vi "Lab Panel V5.10.vi"() -> ()   [LabVIEW 2013] (continued)
              n217 = Bundle By Name(cluster=w250, "TL-1"=w242, "TN-1"=w241, "TL-2"=w240, "TN-2"=w239, "TL -1COUNT"=w247, "TN-1 COUNT"=w247, "TL-2 COUNT"=w247, "TN-2 COUNT"=w247) -> (w248:T9)
              n218 = Bundle(cluster=w245, "Tmp Live"=w240, "Tmp Neut"=w239) -> (w243:T2)  [unwired: 3 in]
              n219 = Bundle(cluster=w246, "Tmp Live"=w242, "Tmp Neut"=w241) -> (w244:T2)  [unwired: 3 in]
              n220 = local write "TEMP LA02"(w248) -> ()
              n221 = local write "SIG LAB02-1"(w244) -> ()
              n222 = local write "SIG LAB02-2"(w243) -> ()
            }
            frame #4 {
              w259 = 0
              n223 = local read "LAB03 TEMP"() -> (w261:T12)
              n224 = Unbundle By Name(w261) -> ("T1 Live"=w254:dbl, "T1 Neut"=w253:dbl, "T2 Live"=w252:dbl, "T2 Neut"=w251:dbl)  [unwired: 2 out]
              n225 = local read "SIG LAB03-1"() -> (w258:T2)
              n226 = local read "SIG LAB03-2"() -> (w257:T2)
              n227 = local read "TEMP LA03"() -> (w262:T9)
              n228 = Bundle By Name(cluster=w262, "TL-1"=w254, "TN-1"=w253, "TL-2"=w252, "TN-2"=w251, "TL -1COUNT"=w259, "TN-1 COUNT"=w259, "TL-2 COUNT"=w259, "TN-2 COUNT"=w259) -> (w260:T9)
              n229 = Bundle(cluster=w257, "Tmp Live"=w252, "Tmp Neut"=w251) -> (w255:T2)  [unwired: 3 in]
              n230 = Bundle(cluster=w258, "Tmp Live"=w254, "Tmp Neut"=w253) -> (w256:T2)  [unwired: 3 in]
              n231 = local write "TEMP LA03"(w260) -> ()
              n232 = local write "SIG LAB03-2"(w255) -> ()
              n233 = local write "SIG LAB03-1"(w256) -> ()
            }
            frame #5 {
              w271 = 0
              n234 = local read "LAB04 TEMP"() -> (w273:T12)
              n235 = Unbundle By Name(w273) -> ("T1 Live"=w266:dbl, "T1 Neut"=w265:dbl, "T2 Live"=w264:dbl, "T2 Neut"=w263:dbl)  [unwired: 2 out]
              n236 = local read "SIG LAB04-2"() -> (w269:T2)
              n237 = local read "SIG LAB04-1"() -> (w270:T2)
              n238 = local read "TEMP LA04"() -> (w274:T9)
              n239 = Bundle By Name(cluster=w274, "TL-1"=w266, "TN-1"=w265, "TL-2"=w264, "TN-2"=w263, "TL -1COUNT"=w271, "TN-1 COUNT"=w271, "TL-2 COUNT"=w271, "TN-2 COUNT"=w271) -> (w272:T9)
              n240 = Bundle(cluster=w269, "Tmp Live"=w264, "Tmp Neut"=w263) -> (w267:T2)  [unwired: 3 in]
              n241 = Bundle(cluster=w270, "Tmp Live"=w266, "Tmp Neut"=w265) -> (w268:T2)  [unwired: 3 in]
              n242 = local write "SIG LAB04-2"(w267) -> ()
              n243 = local write "TEMP LA04"(w272) -> ()
              n244 = local write "SIG LAB04-1"(w268) -> ()
            }
            frame #6 {
              w283 = 0
              n245 = local read "LAB05 TEMP"() -> (w285:T12)
              n246 = Unbundle By Name(w285) -> ("T1 Live"=w278:dbl, "T1 Neut"=w277:dbl, "T2 Live"=w276:dbl, "T2 Neut"=w275:dbl)  [unwired: 2 out]
              n247 = local read "SIG LAB05-2"() -> (w281:T2)
              n248 = local read "SIG LAB05-1"() -> (w282:T2)
              n249 = local read "TEMP LA05"() -> (w286:T9)
              n250 = Bundle By Name(cluster=w286, "TL-1"=w278, "TN-1"=w277, "TL-2"=w276, "TN-2"=w275, "TL -1COUNT"=w283, "TN-1 COUNT"=w283, "TL-2 COUNT"=w283, "TN-2 COUNT"=w283) -> (w284:T9)
              n251 = Bundle(cluster=w281, "Tmp Live"=w276, "Tmp Neut"=w275) -> (w279:T2)  [unwired: 3 in]
              n252 = Bundle(cluster=w282, "Tmp Live"=w278, "Tmp Neut"=w277) -> (w280:T2)  [unwired: 3 in]
              n253 = local write "SIG LAB05-2"(w279) -> ()
              n254 = local write "SIG LAB05-1"(w280) -> ()
              n255 = local write "TEMP LA05"(w284) -> ()
            }
          }
        }
        frame #8 {
          # "enable front panel, all settings done"
          n256 = property on="Tab Control 2" class="TabCtl (strict)"("DisabledEnum"=T16."Enabled" ("Disabled")) -> ()  [unwired: 2 in, 2 out]
          n257 = property on="Tab Control 2" class="TabCtl (strict)"("Value"=0) -> ()  [unwired: 2 in, 2 out]
        }
        frame #9 {
          n258 = property on="Tab Control 2" class="TabCtl (strict)"("Value"=0) -> ()  [unwired: 2 in, 2 out]
        }
      }
    }
    frame #2 {
      n259 = node-c288("loop  delay(mS)") -> (w292:T17)  [unwired: 3 in]
      n260 = timed-loop {
        timing: w292 -> [_]
        timing-out: [_] -> w291
        i -> [w314]
        stop <- "stop" stop-if-true
        n261 = node-c288() -> ()  [unwired: 1 in, 1 out]
        n262 = global write "Global display 1.vi" "stop disp"("stop") -> ()
        n263 = local read "SELECT LAB05-2"() -> (w294:T3)
        n264 = local read "SELECT LAB05-1"() -> (w295:T3)
        n265 = local read "SELECT LAB04-2"() -> (w296:T3)
        n266 = local read "SELECT LAB03-1"() -> (w299:T3)
        n267 = local read "SELECT LAB02-2"() -> (w300:T3)
        n268 = local read "SELECT LAB01-1"() -> (w303:T3)
        n269 = local read "SELECT LAB03-2"() -> (w298:T3)
        n270 = local read "SELECT LAB01-2"() -> (w302:T3)
        n271 = local read "SELECT LAB04-1"() -> (w297:T3)
        n272 = local read "SELECT LAB02-1"() -> (w301:T3)
        n273 = local read "run lab03-2"() -> (w308:bool)
        n274 = local read "run lab04-1"() -> (w307:bool)
        n275 = local read "run lab05-1"() -> (w305:bool)
        n276 = local read "run lab04-2"() -> (w306:bool)
        n277 = local read "run lab05-2"() -> (w304:bool)
        n278 = local read "run lab03-1"() -> (w309:bool)
        n279 = local read "run lab02-2"() -> (w310:bool)
        n280 = local read "run lab02-1"() -> (w311:bool)
        n281 = local read "run lab01-1"() -> (w313:bool)
        n282 = local read "run lab01-2"() -> (w312:bool)
        n283 = stacked-sequence {
          seq-local: [_ w379 _ _ _ _ _ _ _ _ _ _ _ _ _ _ _ _ _ _ _ _ _] -> [_ _ _ _ _ w2480 _ _ _ _ _ _ _ _ _ _ _ _ _ _ _ _ _]
          seq-local: [_ w378 _ _ _ _ _ _ _ _ _ _ _ _ _ _ _ _ _ _ _ _ _] -> [_ _ _ _ _ w2479 _ _ _ _ _ _ _ _ _ _ _ _ _ _ _ _ _]
          seq-local: [_ w365 _ _ _ _ _ _ _ _ _ _ _ _ _ _ _ _ _ _ _ _ _] -> [_ _ _ _ _ w2478 _ _ _ _ _ _ _ _ _ _ _ _ _ _ _ _ _]
          seq-local: [_ w364 _ _ _ _ _ _ _ _ _ _ _ _ _ _ _ _ _ _ _ _ _] -> [_ _ _ _ _ w2477 _ _ _ _ _ _ _ _ _ _ _ _ _ _ _ _ _]
          seq-local: [_ w363 _ _ _ _ _ _ _ _ _ _ _ _ _ _ _ _ _ _ _ _ _] -> [_ _ _ _ _ w2476 _ _ _ _ _ _ _ _ _ _ _ _ _ _ _ _ _]
          seq-local: [_ w362 _ _ _ _ _ _ _ _ _ _ _ _ _ _ _ _ _ _ _ _ _] -> [_ _ _ _ _ w2475 _ _ _ _ _ _ _ _ _ _ _ _ _ _ _ _ _]
          seq-local: [_ w361 _ _ _ _ _ _ _ _ _ _ _ _ _ _ _ _ _ _ _ _ _] -> [_ _ _ _ _ w2474 _ _ _ _ _ _ _ _ _ _ _ _ _ _ _ _ _]
          seq-local: [_ w360 _ _ _ _ _ _ _ _ _ _ _ _ _ _ _ _ _ _ _ _ _] -> [_ _ _ _ _ w2473 _ _ _ _ _ _ _ _ _ _ _ _ _ _ _ _ _]
          seq-local: [_ w359 _ _ _ _ _ _ _ _ _ _ _ _ _ _ _ _ _ _ _ _ _] -> [_ _ _ _ _ w2472 _ _ _ _ _ _ _ _ _ _ _ _ _ _ _ _ _]
          seq-local: [_ w358 _ _ _ _ _ _ _ _ _ _ _ _ _ _ _ _ _ _ _ _ _] -> [_ _ _ _ _ w2471 _ _ _ _ _ _ _ _ _ _ _ _ _ _ _ _ _]
          tunnel: w313 -> [_ _ w395 w643 w2070 w2500 w2815 w3302 _ _ _ _ w3790 _ w4747 _ _ w5034 w5337 w5519 _ _ _]
          tunnel: w312 -> [_ _ w394 w641 w2069 w2499 w2816 w3301 _ _ _ _ w3789 _ w4745 _ _ w5033 w5336 w5517 _ _ _]
          tunnel: w311 -> [_ _ w393 w639 w2068 w2498 w2814 w3300 _ _ _ _ w3788 _ w4743 _ _ w5032 w5335 w5516 _ _ _]
          tunnel: w310 -> [_ _ w392 w637 w2067 w2497 w2813 w3299 _ _ _ _ w3787 _ w4741 _ _ w5031 w5334 w5515 _ _ _]
          tunnel: w309 -> [_ _ w391 w635 w2066 w2496 w2812 w3298 _ _ _ _ w3786 _ w4739 _ _ w5030 w5333 w5514 _ _ _]
          tunnel: w308 -> [_ _ w390 w633 w2065 w2495 w2811 w3297 _ _ _ _ w3785 _ w4737 _ _ w5029 w5332 w5513 _ _ _]
          tunnel: w307 -> [_ _ w389 w631 w2064 w2494 w2810 w3296 _ _ _ _ w3784 _ w4735 _ _ w5028 w5331 w5512 _ _ _]
          tunnel: w306 -> [_ _ w388 w629 w2063 w2493 w2809 w3295 _ _ _ _ w3783 _ w4733 _ _ w5027 w5330 w5511 _ _ _]
          tunnel: w305 -> [_ _ w387 w627 w2062 w2492 w2808 w3294 _ _ _ _ w3782 _ w4731 _ _ w5026 w5329 w5510 _ _ _]
          tunnel: w304 -> [_ _ w386 w625 w2061 w2491 w2807 w3293 _ _ _ _ w3781 _ w4729 _ _ w5025 w5328 w5509 _ _ _]
          tunnel: w303 -> [_ _ _ w642 w2060 w2490 _ _ _ _ _ _ _ _ w4749 _ _ _ _ _ w5863 _ _]
          tunnel: w302 -> [_ _ _ w640 w2059 w2489 _ _ _ _ _ _ _ _ w4744 _ _ _ _ _ w5862 _ _]
          tunnel: w301 -> [_ _ _ w638 w2058 w2488 _ _ _ _ _ _ _ _ w4742 _ _ _ _ _ w5861 _ _]
          tunnel: w300 -> [_ _ _ w636 w2057 w2487 _ _ _ _ _ _ _ _ w4740 _ _ _ _ _ w5860 _ _]
          tunnel: w299 -> [_ _ _ w634 w2056 w2486 _ _ _ _ _ _ _ _ w4738 _ _ _ _ _ w5859 _ _]
          tunnel: w298 -> [_ _ _ w632 w2055 w2485 _ _ _ _ _ _ _ _ w4736 _ _ _ _ _ w5858 _ _]
          tunnel: w297 -> [_ _ _ w630 w2054 w2484 _ _ _ _ _ _ _ _ w4734 _ _ _ _ _ w5857 _ _]
          tunnel: w296 -> [_ _ _ w628 w2053 w2483 _ _ _ _ _ _ _ _ w4732 _ _ _ _ _ w5856 _ _]
          tunnel: w295 -> [_ _ _ w626 w2052 w2482 _ _ _ _ _ _ _ _ w4730 _ _ _ _ _ w5855 _ _]
          tunnel: w294 -> [_ _ _ w624 w2051 w2481 _ _ _ _ _ _ _ _ w4728 _ _ _ _ _ w5854 _ _]
          frame #0 {
            w321 = FALSE
            w326 = 0.5
            # "set up cycle control"
            n284 = local read "jig cycle"() -> (w325:dbl)
            n285 = local read "Amps Fail level"() -> (w319:dbl)
            n286 = Divide(x="JIG ON TIME (S)", y=w326) -> (x/y=→"on loops":dbl)
            n287 = Divide(x="JIG OFF TIME (S)", y=w326) -> (x/y=→"off loops":dbl)
            n288 = global write "Global display 3.vi" "Amps Fail"(w319) -> ()
            n289 = Increment(x=w325) -> (x+1=w324:dbl)
            n290 = local write "TEMP"(w321) -> ()
            n291 = local write "AI"(w321) -> ()
            n292 = local read "Network Directory"() -> (w318:path)
            n293 = local write "jig cycle"(w324) -> ()
            n294 = call "sub vi - check network dir v2.vi"("PATH"=w318) -> ("error"=w317:bool)  [unwired: 10 in]
            n295 = local write "network error"(w317) -> ()
            n296 = global write "Global display 3.vi" "network drive"(w317) -> ()
            n297 = event shown="[1] \"ADMIN\": Value Change" {
              selector: _ -> [_ _]
              dyn-events: _ -> [_ _]
              timeout: 10 -> [_ _]
              event Timeout {
                n298 = event-data() -> ()  [unwired: 1 in, 3 out]
              }
              event "ADMIN": Value Change {
                n299 = event-data() -> ()  [unwired: 1 in, 6 out]
                n300 = stacked-sequence {
                  seq-local: [_ w330 _] -> [_ _ w331]
                  frame #0 {
                    n301 = global write "Global 1.vi" "password"("9949") -> ()
                  }
                  frame #1 {
                    n302 = call "sub vi - password 1.vi"() -> ("RESULT"=w330:bool)  [unwired: 11 in]
                  }
                  frame #2 {
                    w333 = FALSE
                    n303 = property on="Tab Control 2" class="TabCtl (strict)"() -> ("Pages"=w337:refnum<vi>[])  [unwired: 2 in, 2 out]
                    n304 = Select(t=TRUE, s=w331, f=w333) -> (s? t:f=w332:bool)
                    n305 = Index Array(array=w337, index=8) -> (element=w335:refnum<vi>)
                    n306 = property class="Page"(reference=w335, "PageVis"=w332) -> ()  [unwired: 1 in, 2 out]
                    n307 = local write "ADMIN"(w333) -> ()
                  }
                }
              }
            }
          }
          frame #1 {
            w375 = 60.0
            # "convert temperature rise minutes to cycles"
            n308 = local read "SET LAB05-2"() -> (w339:T5)
            n309 = local read "SET LAB05-1"() -> (w341:T5)
            n310 = local read "SET LAB04-2"() -> (w343:T5)
            n311 = local read "SET LAB01-1"() -> (w357:T5)
            n312 = local read "SET LAB01-2"() -> (w355:T5)
            n313 = local read "SET LAB02-2"() -> (w351:T5)
            n314 = local read "SET LAB04-1"() -> (w345:T5)
            n315 = local read "SET LAB03-1"() -> (w349:T5)
            n316 = local read "SET LAB03-2"() -> (w347:T5)
            n317 = local read "SET LAB02-1"() -> (w353:T5)
            n318 = local read "JIG OFF TIME (S)"() -> (w380:dbl)
            n319 = local read "JIG ON TIME (S)"() -> (w381:dbl)
            n320 = Unbundle(w339) -> ("T-RISE mins"=w338:dbl)  [unwired: 4 out]
            n321 = Unbundle(w341) -> ("T-RISE mins"=w340:dbl)  [unwired: 4 out]
            n322 = Unbundle(w357) -> ("T-RISE mins"=w356:dbl)  [unwired: 4 out]
            n323 = Unbundle(w343) -> ("T-RISE mins"=w342:dbl)  [unwired: 4 out]
            n324 = Unbundle(w355) -> ("T-RISE mins"=w354:dbl)  [unwired: 4 out]
            n325 = Unbundle(w353) -> ("T-RISE mins"=w352:dbl)  [unwired: 4 out]
            n326 = Unbundle(w345) -> ("T-RISE mins"=w344:dbl)  [unwired: 4 out]
            n327 = Unbundle(w351) -> ("T-RISE mins"=w350:dbl)  [unwired: 4 out]
            n328 = Unbundle(w347) -> ("T-RISE mins"=w346:dbl)  [unwired: 4 out]
            n329 = Unbundle(w349) -> ("T-RISE mins"=w348:dbl)  [unwired: 4 out]
            n330 = Add(x=w381, y=w380) -> (x+y=w374:dbl)
            n331 = Multiply(x=w375, y=w346) -> (x*y=w370:dbl)
            n332 = Multiply(x=w375, y=w344) -> (x*y=w369:dbl)
            n333 = Multiply(x=w375, y=w342) -> (x*y=w368:dbl)
            n334 = Multiply(x=w375, y=w340) -> (x*y=w367:dbl)
            n335 = Multiply(x=w375, y=w338) -> (x*y=w366:dbl)
            n336 = Multiply(x=w375, y=w354) -> (x*y=w376:dbl)
            n337 = Multiply(x=w375, y=w348) -> (x*y=w371:dbl)
            n338 = Multiply(x=w375, y=w356) -> (x*y=w377:dbl)
            n339 = Multiply(x=w375, y=w352) -> (x*y=w373:dbl)
            n340 = Multiply(x=w375, y=w350) -> (x*y=w372:dbl)
            n341 = Divide(x=w367, y=w374) -> (x/y=w359:dbl)
            n342 = Divide(x=w368, y=w374) -> (x/y=w360:dbl)
            n343 = Divide(x=w369, y=w374) -> (x/y=w361:dbl)
            n344 = Divide(x=w366, y=w374) -> (x/y=w358:dbl)
            n345 = Divide(x=w371, y=w374) -> (x/y=w363:dbl)
            n346 = Divide(x=w377, y=w374) -> (x/y=w379:dbl)
            n347 = Divide(x=w376, y=w374) -> (x/y=w378:dbl)
            n348 = Divide(x=w373, y=w374) -> (x/y=w365:dbl)
            n349 = Divide(x=w372, y=w374) -> (x/y=w364:dbl)
            n350 = Divide(x=w370, y=w374) -> (x/y=w362:dbl)
          }
          frame #2 {
            # "control cycle loops"
            n351 = local read "JIG OFF TIME (S)"() -> (w384:dbl)
            n352 = local read "JIG ON TIME (S)"() -> (w383:dbl)
            n353 = local read "jig cycle"() -> (w397:dbl)
            n354 = local read "on loops"() -> (w399:dbl)
            n355 = local read "off loops"() -> (w398:dbl)
            n356 = Add(x=w384, y=w383) -> (x+y=w382:dbl)
            n357 = Add(x=w399, y=w398) -> (x+y=w385:dbl)
            n358 = Greater Or Equal?(x=w397, y=w385) -> (x >= y?=w396:bool)
            n359 = case shown="True" w396 {
              tunnel: w395 -> [_ w433]
              tunnel: w394 -> [_ w432]
              tunnel: w393 -> [_ w431]
              tunnel: w392 -> [_ w430]
              tunnel: w391 -> [_ w429]
              tunnel: w390 -> [_ w428]
              tunnel: w389 -> [_ w427]
              tunnel: w388 -> [_ w426]
              tunnel: w387 -> [_ w425]
              tunnel: w386 -> [_ w424]
              tunnel: w382 -> [_ w423]
              frame False {
              }
              frame True {
                # "increment cycle value and convert cycles to minutes for temp rise"
                n360 = stacked-sequence {
                  frame #0 {
                    n361 = local read "Panel #"() -> (w436:dbl)
                    n362 = Increment(x=w436) -> (x+1=w435:dbl)
                    n363 = local write "Panel #"(w435) -> ()
                  }
                  frame #1 {
                    n364 = local read "Panel #"() -> (w437:dbl)
                    n365 = Greater?(x=w437, y=5) -> (0:w439:bool)
                    n366 = case shown="True" w439 {
                      frame False {
                      }
                      frame True {
                        n367 = local write "Panel #"(1) -> ()
                      }
                    }
                  }
                }
                n368 = local read "JIG RELAY CYCLES"() -> (w422:T8)
                n369 = local read "Panel #"() -> (→"Tp Ut":dbl)
                n370 = Unbundle By Name(w422) -> ("LAB01-1"=w420:dbl, "LAB01-2"=w418:dbl, "LAB02-1"=w416:dbl, "LAB02-2"=w414:dbl, "LAB03-1"=w412:dbl, "LAB03-2"=w410:dbl, "LAB04-1"=w408:dbl, "LAB04-2"=w406:dbl, "LAB05-1"=w404:dbl, "LAB05-2"=w402:dbl)
                n371 = stacked-sequence {
                  tunnel: w433 -> [w451 _ _ _ _ _ _ _ _ _]
                  tunnel: w432 -> [_ w468 _ _ _ _ _ _ _ _]
                  tunnel: w431 -> [_ _ w485 _ _ _ _ _ _ _]
                  tunnel: w430 -> [_ _ _ w502 _ _ _ _ _ _]
                  tunnel: w429 -> [_ _ _ _ w519 _ _ _ _ _]
                  tunnel: w428 -> [_ _ _ _ _ w536 _ _ _ _]
                  tunnel: w427 -> [_ _ _ _ _ _ w553 _ _ _]
                  tunnel: w426 -> [_ _ _ _ _ _ _ w570 _ _]
                  tunnel: w425 -> [_ _ _ _ _ _ _ _ w587 _]
                  tunnel: w424 -> [_ _ _ _ _ _ _ _ _ w604]
                  tunnel: w423 -> [w448 w465 w482 w499 w516 w533 w550 w567 w584 w601]
                  tunnel: w420 -> [w442 _ _ _ _ _ _ _ _ _]
                  tunnel: [w441 _ _ _ _ _ _ _ _ _] -> w419
                  tunnel: w418 -> [_ w459 _ _ _ _ _ _ _ _]
                  tunnel: [_ w458 _ _ _ _ _ _ _ _] -> w417
                  tunnel: w416 -> [_ _ w476 _ _ _ _ _ _ _]
                  tunnel: [_ _ w475 _ _ _ _ _ _ _] -> w415
                  tunnel: w414 -> [_ _ _ w493 _ _ _ _ _ _]
                  tunnel: [_ _ _ w492 _ _ _ _ _ _] -> w413
                  tunnel: w412 -> [_ _ _ _ w510 _ _ _ _ _]
                  tunnel: [_ _ _ _ w509 _ _ _ _ _] -> w411
                  tunnel: w410 -> [_ _ _ _ _ w527 _ _ _ _]
                  tunnel: [_ _ _ _ _ w526 _ _ _ _] -> w409
                  tunnel: w408 -> [_ _ _ _ _ _ w544 _ _ _]
                  tunnel: [_ _ _ _ _ _ w543 _ _ _] -> w407
                  tunnel: w406 -> [_ _ _ _ _ _ _ w561 _ _]
                  tunnel: [_ _ _ _ _ _ _ w560 _ _] -> w405
                  tunnel: w404 -> [_ _ _ _ _ _ _ _ w578 _]
                  tunnel: [_ _ _ _ _ _ _ _ w577 _] -> w403
                  tunnel: w402 -> [_ _ _ _ _ _ _ _ _ w595]
                  tunnel: [_ _ _ _ _ _ _ _ _ w594] -> w401
                  frame #0 {
                    n372 = local read "DISP LAB01-1"() -> (w446:T4)
                    n373 = Unbundle(w446) -> ("CYCLE"=w447:dbl)  [unwired: 2 out]
                    n374 = case shown="True" w451 {
                      tunnel: w447 -> [w453 w457]
                      tunnel: [w453 w456] -> w445
                      tunnel: w442 -> [w452 w455]
                      tunnel: [w452 w454] -> w441
                      frame False {
                      }
                      frame True {
                        n375 = Increment(x=w455) -> (x+1=w454:dbl)
                        n376 = Increment(x=w457) -> (x+1=w456:dbl)
                      }
                    }
                    n377 = Multiply(x=w445, y=w448) -> (x*y=w449:dbl)
                    n378 = Divide(x=w449, y=60.0) -> (x/y=w444:dbl)
                    n379 = Bundle(cluster=w446, "CYCLE"=w445, "MINS"=w444) -> (w443:T4)  [unwired: 1 in]
                    n380 = local write "DISP LAB01-1"(w443) -> ()
                  }
                  frame #1 {
                    n381 = local read "DISP LAB01-2"() -> (w463:T4)
                    n382 = Unbundle(w463) -> ("CYCLE"=w464:dbl)  [unwired: 2 out]
                    n383 = case shown="True" w468 {
                      tunnel: w464 -> [w470 w474]
                      tunnel: [w470 w473] -> w461
                      tunnel: w459 -> [w469 w472]
                      tunnel: [w469 w471] -> w458
                      frame False {
                      }
                      frame True {
                        n384 = Increment(x=w472) -> (x+1=w471:dbl)
                        n385 = Increment(x=w474) -> (x+1=w473:dbl)
                      }
                    }
                    n386 = Multiply(x=w461, y=w465) -> (x*y=w466:dbl)
                    n387 = Divide(x=w466, y=60.0) -> (x/y=w460:dbl)
                    n388 = Bundle(cluster=w463, "CYCLE"=w461, "MINS"=w460) -> (w462:T4)  [unwired: 1 in]
                    n389 = local write "DISP LAB01-2"(w462) -> ()
                  }
                  frame #2 {
                    n390 = local read "DISP LAB02-1"() -> (w480:T4)
                    n391 = Unbundle(w480) -> ("CYCLE"=w481:dbl)  [unwired: 2 out]
                    n392 = case shown="True" w485 {
                      tunnel: [w487 w491] -> w478
                      tunnel: w481 -> [w487 w490]
                      tunnel: w476 -> [w486 w489]
                      tunnel: [w486 w488] -> w475
                      frame False {
                      }
                      frame True {
                        n393 = Increment(x=w489) -> (x+1=w488:dbl)
                        n394 = Increment(x=w490) -> (x+1=w491:dbl)
                      }
                    }
                    n395 = Multiply(x=w478, y=w482) -> (x*y=w483:dbl)
                    n396 = Divide(x=w483, y=60.0) -> (x/y=w477:dbl)
                    n397 = Bundle(cluster=w480, "CYCLE"=w478, "MINS"=w477) -> (w479:T4)  [unwired: 1 in]
                    n398 = local write "DISP LAB02-1"(w479) -> ()
                  }
                  frame #3 {
                    n399 = local read "DISP LAB02-2"() -> (w497:T4)
                    n400 = Unbundle(w497) -> ("CYCLE"=w498:dbl)  [unwired: 2 out]
                    n401 = case shown="True" w502 {
                      tunnel: [w504 w508] -> w496
                      tunnel: w498 -> [w504 w507]
                      tunnel: w493 -> [w503 w506]
                      tunnel: [w503 w505] -> w492
                      frame False {
                      }
                      frame True {
                        n402 = Increment(x=w506) -> (x+1=w505:dbl)
                        n403 = Increment(x=w507) -> (x+1=w508:dbl)
                      }
                    }
                    n404 = Multiply(x=w496, y=w499) -> (x*y=w500:dbl)
                    n405 = Divide(x=w500, y=60.0) -> (x/y=w495:dbl)
                    n406 = Bundle(cluster=w497, "CYCLE"=w496, "MINS"=w495) -> (w494:T4)  [unwired: 1 in]
                    n407 = local write "DISP LAB02-2"(w494) -> ()
                  }
                  frame #4 {
                    n408 = local read "DISP LAB03-1"() -> (w514:T4)
                    n409 = Unbundle(w514) -> ("CYCLE"=w515:dbl)  [unwired: 2 out]
                    n410 = case shown="True" w519 {
                      tunnel: [w521 w525] -> w511
                      tunnel: w515 -> [w521 w524]
                      tunnel: w510 -> [w520 w523]
                      tunnel: [w520 w522] -> w509
                      frame False {
                      }
                      frame True {
                        n411 = Increment(x=w523) -> (x+1=w522:dbl)
                        n412 = Increment(x=w524) -> (x+1=w525:dbl)
                      }
                    }
                    n413 = Multiply(x=w511, y=w516) -> (x*y=w517:dbl)
                    n414 = Divide(x=w517, y=60.0) -> (x/y=w512:dbl)
                    n415 = Bundle(cluster=w514, "CYCLE"=w511, "MINS"=w512) -> (w513:T4)  [unwired: 1 in]
                    n416 = local write "DISP LAB03-1"(w513) -> ()
                  }
                  frame #5 {
                    n417 = local read "DISP LAB03-2"() -> (w531:T4)
                    n418 = Unbundle(w531) -> ("CYCLE"=w532:dbl)  [unwired: 2 out]
                    n419 = case shown="True" w536 {
                      tunnel: [w538 w542] -> w530
                      tunnel: w532 -> [w538 w541]
                      tunnel: w527 -> [w537 w540]
                      tunnel: [w537 w539] -> w526
                      frame False {
                      }
                      frame True {
                        n420 = Increment(x=w540) -> (x+1=w539:dbl)
                        n421 = Increment(x=w541) -> (x+1=w542:dbl)
                      }
                    }
                    n422 = Multiply(x=w530, y=w533) -> (x*y=w534:dbl)
                    n423 = Divide(x=w534, y=60.0) -> (x/y=w529:dbl)
                    n424 = Bundle(cluster=w531, "CYCLE"=w530, "MINS"=w529) -> (w528:T4)  [unwired: 1 in]
                    n425 = local write "DISP LAB03-2"(w528) -> ()
                  }
                  frame #6 {
                    n426 = local read "DISP LAB04-1"() -> (w548:T4)
                    n427 = Unbundle(w548) -> ("CYCLE"=w549:dbl)  [unwired: 2 out]
                    n428 = case shown="True" w553 {
                      tunnel: [w555 w559] -> w546
                      tunnel: w549 -> [w555 w558]
                      tunnel: w544 -> [w554 w557]
                      tunnel: [w554 w556] -> w543
                      frame False {
                      }
                      frame True {
                        n429 = Increment(x=w557) -> (x+1=w556:dbl)
                        n430 = Increment(x=w558) -> (x+1=w559:dbl)
                      }
                    }
                    n431 = Multiply(x=w546, y=w550) -> (x*y=w551:dbl)
                    n432 = Divide(x=w551, y=60.0) -> (x/y=w545:dbl)
                    n433 = Bundle(cluster=w548, "CYCLE"=w546, "MINS"=w545) -> (w547:T4)  [unwired: 1 in]
                    n434 = local write "DISP LAB04-1"(w547) -> ()
                  }
                  frame #7 {
                    n435 = local read "DISP LAB04-2"() -> (w565:T4)
                    n436 = Unbundle(w565) -> ("CYCLE"=w566:dbl)  [unwired: 2 out]
                    n437 = case shown="True" w570 {
                      tunnel: [w572 w576] -> w563
                      tunnel: w566 -> [w572 w575]
                      tunnel: w561 -> [w571 w574]
                      tunnel: [w571 w573] -> w560
                      frame False {
                      }
                      frame True {
                        n438 = Increment(x=w574) -> (x+1=w573:dbl)
                        n439 = Increment(x=w575) -> (x+1=w576:dbl)
                      }
                    }
                    n440 = Multiply(x=w563, y=w567) -> (x*y=w569:dbl)
                    n441 = Divide(x=w569, y=60.0) -> (x/y=w562:dbl)
                    n442 = Bundle(cluster=w565, "CYCLE"=w563, "MINS"=w562) -> (w564:T4)  [unwired: 1 in]
                    n443 = local write "DISP LAB04-2"(w564) -> ()
                  }
                  frame #8 {
                    n444 = local read "DISP LAB05-1"() -> (w582:T4)
                    n445 = Unbundle(w582) -> ("CYCLE"=w583:dbl)  [unwired: 2 out]
                    n446 = case shown="True" w587 {
                      tunnel: [w589 w593] -> w580
                      tunnel: w583 -> [w589 w592]
                      tunnel: w578 -> [w588 w591]
                      tunnel: [w588 w590] -> w577
                      frame False {
                      }
                      frame True {
                        n447 = Increment(x=w591) -> (x+1=w590:dbl)
                        n448 = Increment(x=w592) -> (x+1=w593:dbl)
                      }
                    }
                    n449 = Multiply(x=w580, y=w584) -> (x*y=w585:dbl)
                    n450 = Divide(x=w585, y=60.0) -> (x/y=w579:dbl)
                    n451 = Bundle(cluster=w582, "CYCLE"=w580, "MINS"=w579) -> (w581:T4)  [unwired: 1 in]
                    n452 = local write "DISP LAB05-1"(w581) -> ()
                  }
                  frame #9 {
                    n453 = local read "DISP LAB05-2"() -> (w600:T4)
                    n454 = Unbundle(w600) -> ("CYCLE"=w599:dbl)  [unwired: 2 out]
                    n455 = case shown="True" w604 {
                      tunnel: [w606 w610] -> w598
                      tunnel: w599 -> [w606 w609]
                      tunnel: w595 -> [w605 w608]
                      tunnel: [w605 w607] -> w594
                      frame False {
                      }
                      frame True {
                        n456 = Increment(x=w608) -> (x+1=w607:dbl)
                        n457 = Increment(x=w609) -> (x+1=w610:dbl)
                      }
                    }
                    n458 = Multiply(x=w598, y=w601) -> (x*y=w602:dbl)
                    n459 = Divide(x=w602, y=60.0) -> (x/y=w597:dbl)
                    n460 = Bundle(cluster=w600, "CYCLE"=w598, "MINS"=w597) -> (w596:T4)  [unwired: 1 in]
                    n461 = local write "DISP LAB05-2"(w596) -> ()
                  }
                }
                n462 = local write "jig cycle"(0) -> ()
                n463 = Bundle By Name(cluster=w422, "LAB01-1"=w419, "LAB01-2"=w417, "LAB02-1"=w415, "LAB02-2"=w413, "LAB03-1"=w411, "LAB03-2"=w409, "LAB04-1"=w407, "LAB04-2"=w405, "LAB05-1"=w403, "LAB05-2"=w401) -> (w421:T8)
                n464 = local write "JIG RELAY CYCLES"(w421) -> ()
              }
            }
          }
          frame #3 {
            # "START & STOP test RUN switch change, start test if true and stop test if false"
            n465 = Get Date/Time In Seconds() -> (seconds since 1Jan1904=w622:timestamp)
            n466 = local read "C drive data root dir"() -> (w615:path)
            n467 = Format Date/Time String(time format string (%c)="%b\\%a%d", seconds (now)=w622) -> (date/time string=w646:string)  [unwired: 1 in]
            n468 = Format Date/Time String(time format string (%c)="%H%M", seconds (now)=w622) -> (date/time string=w644:string)  [unwired: 1 in]
            n469 = Format Date/Time String(time format string (%c)="LabPanel%Y", seconds (now)=w622) -> (date/time string=w621:string)  [unwired: 1 in]
            n470 = Path To String(path=w615) -> (string=w618:string)
            n471 = global write "Global 1.vi" "C drive root path"(w615) -> ()
            n472 = local read "Ref deg C"() -> (w611:dbl)
            n473 = Concatenate Strings(w618, "\\") -> (w616:string)
            n474 = event shown="[1] \"RUN LAB01-1\": Value Change" {
              selector: _ -> [_ _ _ _ _ _ _ _ _ _ _]
              dyn-events: _ -> [_ _ _ _ _ _ _ _ _ _ _]
              timeout: 10 -> [_ _ _ _ _ _ _ _ _ _ _]
              tunnel: w616 -> [_ w659 w799 w940 w1080 w1220 w1360 w1500 w1640 w1780 w1921]
              tunnel: w646 -> [_ w658 w798 w939 w1079 w1219 w1359 w1499 w1639 w1779 w1920]
              tunnel: w644 -> [_ w656 w797 w938 w1078 w1218 w1358 w1498 w1638 w1778 w1919]
              tunnel: w642 -> [_ w657 _ _ _ _ _ _ _ _ _]
              tunnel: w643 -> [_ _ _ _ _ _ _ _ _ _ _]
              tunnel: w641 -> [_ _ _ _ _ _ _ _ _ _ _]
              tunnel: w640 -> [_ _ w796 _ _ _ _ _ _ _ _]
              tunnel: w639 -> [_ _ _ _ _ _ _ _ _ _ _]
              tunnel: w638 -> [_ _ _ w937 _ _ _ _ _ _ _]
              tunnel: w637 -> [_ _ _ _ _ _ _ _ _ _ _]
              tunnel: w636 -> [_ _ _ _ w1077 _ _ _ _ _ _]
              tunnel: w635 -> [_ _ _ _ _ _ _ _ _ _ _]
              tunnel: w634 -> [_ _ _ _ _ w1217 _ _ _ _ _]
              tunnel: w633 -> [_ _ _ _ _ _ _ _ _ _ _]
              tunnel: w632 -> [_ _ _ _ _ _ w1357 _ _ _ _]
              tunnel: w631 -> [_ _ _ _ _ _ _ _ _ _ _]
              tunnel: w630 -> [_ _ _ _ _ _ _ w1497 _ _ _]
              tunnel: w629 -> [_ _ _ _ _ _ _ _ _ _ _]
              tunnel: w628 -> [_ _ _ _ _ _ _ _ w1637 _ _]
              tunnel: w627 -> [_ _ _ _ _ _ _ _ _ _ _]
              tunnel: w626 -> [_ _ _ _ _ _ _ _ _ w1777 _]
              tunnel: w625 -> [_ _ _ _ _ _ _ _ _ _ _]
              tunnel: w624 -> [_ _ _ _ _ _ _ _ _ _ w1918]
              tunnel: w621 -> [_ w655 w795 w936 w1076 w1216 w1356 w1496 w1636 w1776 w1917]
              tunnel: [_ w654 w794 w935 w1075 w1215 w1355 w1495 w1635 w1775 w1916] -> w619
              tunnel: "RESET CYCLES TO ZERO?" -> [_ w653 w792 w933 w1073 w1213 w1353 w1493 w1633 w1773 w1914]
              tunnel: "YES" -> [_ w652 w791 w932 w1072 w1212 w1352 w1492 w1632 w1772 w1913]
              tunnel: "NO" -> [_ w651 w790 w931 w1071 w1211 w1351 w1491 w1631 w1771 w1912]
              tunnel: w611 -> [_ w648 w789 w929 w1070 w1210 w1350 w1490 w1630 w1770 w1910]
              event Timeout {
                n475 = event-data() -> ()  [unwired: 1 in, 3 out]
              }
              event "RUN LAB01-1": Value Change {
                n476 = event-data() -> ("NewVal"=w649:bool)  [unwired: 1 in, 5 out]
                n477 = local read "SIG LAB01-1"() -> (w650:T2)
                n478 = local write "run lab01-1"(w649) -> ()
                n479 = case shown="True" w649 {
                  tunnel: w659 -> [_ w697]
                  tunnel: w658 -> [_ w696]
                  tunnel: w657 -> [w661 w695]
                  tunnel: w656 -> [_ w694]
                  tunnel: w655 -> [_ w693]
                  tunnel: [w660 w692] -> w654
                  tunnel: w653 -> [_ w691]
                  tunnel: w652 -> [_ w690]
                  tunnel: w651 -> [_ w689]
                  tunnel: w650 -> [_ w688]
                  tunnel: w648 -> [_ w687]
                  frame False {
                    # "stop test"
                    n480 = stacked-sequence {
                      tunnel: w661 -> [_ w673 _]
                      tunnel: [_ w665 _] -> w660
                      frame #0 {
                        n481 = local read "DISP LAB01-1"() -> (w664:T4)
                        n482 = Bundle(cluster=w664, "STATUS"="STOP") -> (w662:T4)  [unwired: 2 in]
                        n483 = local write "DISP LAB01-1"(w662) -> ()
                      }
                      frame #1 {
                        n484 = local read "DISP LAB01-1"() -> (w672:T4)
                        n485 = Unbundle(w672) -> ("CYCLE"=w670:dbl, "MINS"=w671:dbl)  [unwired: 1 out]
                        n486 = case shown="\"CYCLE TEST\"" w673 {
                          tunnel: w671 -> [_ _ w680]
                          tunnel: w670 -> [w678 w679 _]
                          tunnel: [w678 w679 w680] -> w669
                          frame "CHART TEST", Default {
                          }
                          frame "CYCLE TEST" {
                          }
                          frame "T-RISE TEST" {
                          }
                        }
                        n487 = local read "TDMS LAB01-1"() -> (w677:refnum<k34>)
                        n488 = Build Array("STOPPED") -> (w674:string[])
                        n489 = Build Array(w669) -> (w668:dbl[])
                        n490 = TDMS Write(0:w677, 5:"TEST RESULT", 7:w674, 9:w668) -> (4:w666:refnum<k34>, 15:w667:errorcluster)  [unwired: 2 in, 2 out]
                        n491 = TDMS Close(8:w667, 11:w666) -> (0:w665:errorcluster)  [unwired: 1 out]
                      }
                      frame #2 {
                        n492 = stacked-sequence {
                          tunnel: "LAB01-1" -> [w683 w685]
                          frame #0 {
                            n493 = call "sub vi - defrag tdms v1.vi"("panel id"=w683) -> ("error out"=w682:errorcluster)  [unwired: 10 in]
                            n494 = local write "data file error"(w682) -> ()
                          }
                          frame #1 {
                            n495 = call "Save data file (stop) v3.vi"("panel id"=w685) -> ("network file save error"=w684:errorcluster)  [unwired: 9 in, 1 out]
                            n496 = local write "RESULT LAB01-1"(FALSE) -> ()
                            n497 = local write "data file error"(w684) -> ()
                          }
                        }
                      }
                    }
                  }
                  frame True {
                    n498 = stacked-sequence {
                      seq-local: [w699 _] -> [_ w703]
                      tunnel: w697 -> [_ w713]
                      tunnel: w696 -> [_ w712]
                      tunnel: w695 -> [_ w711]
                      tunnel: w694 -> [_ w710]
                      tunnel: w693 -> [_ w709]
                      tunnel: [_ w708] -> w692
                      tunnel: w691 -> [_ w707]
                      tunnel: w690 -> [_ w706]
                      tunnel: w689 -> [_ w705]
                      tunnel: w688 -> [w701 w704]
                      tunnel: w687 -> [_ w702]
                      frame #0 {
                        n499 = Unbundle(w701) -> ("AMPS"=w700:dbl)  [unwired: 4 out]
                        n500 = call "Check For Amps on v1.vi"("ID"="LAB01-1", "amps"=w700) -> ("amps"=w699:bool)  [unwired: 9 in]
                      }
                      frame #1 {
                        n501 = case shown="True" w703 {
                          tunnel: w713 -> [_ w726]
                          tunnel: w712 -> [_ w725]
                          tunnel: w711 -> [_ w724]
                          tunnel: w710 -> [_ w723]
                          tunnel: w709 -> [_ w722]
                          tunnel: [errorcluster {"status"=FALSE, "code"=0, "source"=""} ("error out") w721] -> w708
                          tunnel: w707 -> [_ w720]
                          tunnel: w706 -> [_ w719]
                          tunnel: w705 -> [_ w718]
                          tunnel: w704 -> [_ w717]
                          tunnel: w702 -> [_ w716]
                          frame False {
                            w714 = FALSE
                            n502 = local write "RUN LAB01-1"(w714) -> ()
                            n503 = local write "run lab01-1"(w714) -> ()
                          }
                          frame True {
                            n504 = stacked-sequence {
                              seq-local: [w727 _ _ _ _] -> [_ w748 _ _ _]
                              tunnel: w726 -> [w732 _ _ _ _]
                              tunnel: w725 -> [w728 _ _ _ _]
                              tunnel: w724 -> [w742 _ _ _ _]
                              tunnel: w723 -> [w735 _ _ _ _]
                              tunnel: w722 -> [w730 _ _ _ _]
                              tunnel: [_ w749 _ _ _] -> w721
                              tunnel: w720 -> [_ _ _ w770 _]
                              tunnel: w719 -> [_ _ _ w780 _]
                              tunnel: w718 -> [_ _ _ w779 _]
                              tunnel: w717 -> [_ _ _ _ _]
                              tunnel: w716 -> [_ _ _ _ w786]
                              frame #0 {
                                w729 = "\\"
                                n505 = case shown="\"CHART TEST\", Default" w742 {
                                tunnel: ["L01-1-CHART TEST-" "L01-1-CYCLE TEST-" "L01-1-T-RISE TEST-"] -> w738
                                frame "CHART TEST", Default {
                                }
                                frame "CYCLE TEST" {
                                }
                                frame "T-RISE TEST" {
                                }
                                }
                                n506 = local read "SET LAB01-1"() -> (w737:T5)
                                n507 = Unbundle(w737) -> ("DESCRIPTION"=w736:string)  [unwired: 4 out]
                                n508 = Concatenate Strings(w732, "\\", w730, w729, w728, w729) -> (w739:string)
                                n509 = String To Path(string=w739) -> (path=w741:path)
                                n510 = Concatenate Strings(w739, w738, w736, "-", w735, ".tdms") -> (w727:string)
                                n511 = Create Folder(path (use dialog)=w741) -> (error out=w740:errorcluster)  [unwired: 2 in, 2 out]
                                n512 = call <vilib>:"Clear Errors.vi"("error in (no error)"=w740) -> ()  [unwired: 6 in, 1 out]
                                n513 = global write "Global 1.vi" "LAB01-1 FILE"(w727) -> ()
                              }
                              frame #1 {
                                (unwired) FALSE
                                n514 = String To Path(string=w748) -> (path=w746:path)
                                n515 = TDMS Open(6:FALSE, 10:T20."create or replace" ("operation (0:open)"), 11:w746) -> (0:w749:errorcluster, 3:→"TDMS LAB01-1":refnum<k34>)  [unwired: 4 in]
                              }
                              frame #2 {
                                n516 = local read "TDMS LAB01-1"() -> (w768:refnum<k34>)
                                n517 = local read "SET LAB01-1"() -> (w757:T5)
                                n518 = Build Array("Testers Name", "Description", "Set Test Cycles", "T-Rise minutes", "T-Rise Deg C") -> (w758:string[])
                                n519 = Unbundle(w757) -> ("NAME"=w756:string, "DESCRIPTION"=w755:string, "CYCLES"=w754:dbl, "T-RISE mins"=w753:dbl, "T-RISE deg C"=w752:dbl)
                                n520 = Number To Decimal String(number=w754) -> (decimal integer string=w767:string)  [unwired: 1 in]
                                n521 = Number To Decimal String(number=w753) -> (decimal integer string=w766:string)  [unwired: 1 in]
                                n522 = Number To Decimal String(number=w752) -> (decimal integer string=w765:string)  [unwired: 1 in]
                                n523 = Build Array(w756, w755, w767, w766, w765) -> (w764:string[])
                                n524 = TDMS Set Properties(5:w764, 7:w758, 11:w768) -> ()  [unwired: 3 in, 4 out]
                              }
                              frame #3 {
                                n525 = local read "DISP LAB01-1"() -> (w778:T4)
                                n526 = Concatenate Strings("LAB01-1  ", w770) -> (w769:string)
                                n527 = Two Button Dialog(message=w769, 1:w779, 2:w780) -> (T button?=w772:bool)
                                n528 = case shown="True" w772 {
                                tunnel: w778 -> [w783 w784]
                                tunnel: [w783 w784] -> w777
                                tunnel: [w782 w785] -> w776
                                tunnel: [w781 w785] -> w775
                                frame False {
                                n529 = Unbundle(w783) -> ("CYCLE"=w782:dbl, "MINS"=w781:dbl)  [unwired: 1 out]
                                }
                                frame True {
                                w785 = 0.0
                                }
                                }
                                n530 = Bundle(cluster=w777, "CYCLE"=w776, "MINS"=w775, "STATUS"="RUN") -> (w774:T4)
                                n531 = local write "DISP LAB01-1"(w774) -> ()
                              }
                              frame #4 {
                                n532 = local read "TEMP START LAB01-1"() -> (w788:cluster{"TL":dbl, "TN":dbl})
                                n533 = Bundle(cluster=w788, "TL"=w786, "TN"=w786) -> (w787:cluster{"TL":dbl, "TN":dbl})
                                n534 = local write "TEMP START LAB01-1"(w787) -> ()
                              }
                            }
                          }
                        }
                      }
                    }
                  }
                }
              }
              event "RUN LAB01-2": Value Change {
                n535 = event-data() -> ("NewVal"=w793:bool)  [unwired: 1 in, 5 out]
                n536 = local write "run lab01-2"(w793) -> ()
                n537 = case shown="True" w793 {
                  tunnel: w799 -> [_ w837]
                  tunnel: w798 -> [_ w836]
                  tunnel: w796 -> [w801 w835]
                  tunnel: w797 -> [_ w834]
                  tunnel: w795 -> [_ w833]
                  tunnel: [w800 w832] -> w794
                  tunnel: w792 -> [_ w831]
                  tunnel: w791 -> [_ w830]
                  tunnel: w790 -> [_ w829]
                  tunnel: w789 -> [_ w827]
                  frame False {
                    # "stop test"
                    n538 = stacked-sequence {
                      tunnel: w801 -> [w810 _]
                      tunnel: [w802 _] -> w800
                      frame #0 {
                        n539 = local read "DISP LAB01-2"() -> (w809:T4)
                        n540 = Unbundle(w809) -> ("CYCLE"=w807:dbl, "MINS"=w808:dbl)  [unwired: 1 out]
                        n541 = case shown="\"CHART TEST\", Default" w810 {
                          tunnel: w808 -> [_ _ w817]
                          tunnel: w807 -> [w815 w816 _]
                          tunnel: [w815 w816 w817] -> w806
                          frame "CHART TEST", Default {
                          }
                          frame "CYCLE TEST" {
                          }
                          frame "T-RISE TEST" {
                          }
                        }
                        n542 = local read "TDMS LAB01-2"() -> (w814:refnum<k34>)
                        n543 = Build Array("STOPPED") -> (w811:string[])
                        n544 = Build Array(w806) -> (w805:dbl[])
                        n545 = TDMS Write(0:w814, 5:"TEST RESULT", 7:w811, 9:w805) -> (4:w803:refnum<k34>, 15:w804:errorcluster)  [unwired: 2 in, 2 out]
                        n546 = TDMS Close(8:w804, 11:w803) -> (0:w802:errorcluster)  [unwired: 1 out]
                      }
                      frame #1 {
                        n547 = local read "DISP LAB01-2"() -> (w821:T4)
                        n548 = stacked-sequence {
                          tunnel: "LAB01-2" -> [w823 w825]
                          frame #0 {
                            n549 = call "sub vi - defrag tdms v1.vi"("panel id"=w823) -> ("error out"=w822:errorcluster)  [unwired: 10 in]
                            n550 = local write "data file error"(w822) -> ()
                          }
                          frame #1 {
                            n551 = call "Save data file (stop) v3.vi"("panel id"=w825) -> ("network file save error"=w824:errorcluster)  [unwired: 9 in, 1 out]
                            n552 = local write "RESULT LAB01-2"(FALSE) -> ()
                            n553 = local write "data file error"(w824) -> ()
                          }
                        }
                        n554 = Bundle(cluster=w821, "STATUS"="STOP") -> (w819:T4)  [unwired: 2 in]
                        n555 = local write "DISP LAB01-2"(w819) -> ()
                      }
                    }
                  }
                  frame True {
                    n556 = local read "SIG LAB01-2"() -> (w828:T2)
                    n557 = stacked-sequence {
                      seq-local: [w839 _] -> [_ w843]
                      tunnel: w837 -> [_ w853]
                      tunnel: w836 -> [_ w852]
                      tunnel: w835 -> [_ w851]
                      tunnel: w834 -> [_ w850]
                      tunnel: w833 -> [_ w849]
                      tunnel: [_ w848] -> w832
                      tunnel: w831 -> [_ w847]
                      tunnel: w830 -> [_ w846]
                      tunnel: w829 -> [_ w845]
                      tunnel: w828 -> [w838 w844]
                      tunnel: w827 -> [_ w842]
                      frame #0 {
                        n558 = Unbundle(w838) -> ("AMPS"=w841:dbl)  [unwired: 4 out]
                        n559 = call "Check For Amps on v1.vi"("ID"="LAB01-2", "amps"=w841) -> ("amps"=w839:bool)  [unwired: 9 in]
                      }
                      frame #1 {
                        n560 = case shown="True" w843 {
                          tunnel: w853 -> [_ w866]
                          tunnel: w852 -> [_ w865]
                          tunnel: w851 -> [_ w864]
                          tunnel: w850 -> [_ w863]
                          tunnel: w849 -> [_ w862]
                          tunnel: [errorcluster {"status"=FALSE, "code"=0, "source"=""} ("error out") w861] -> w848
                          tunnel: w847 -> [_ w860]
                          tunnel: w846 -> [_ w859]
                          tunnel: w845 -> [_ w858]
                          tunnel: w844 -> [_ w857]
                          tunnel: w842 -> [_ w856]
                          frame False {
                            w854 = FALSE
                            n561 = local write "RUN LAB01-2"(w854) -> ()
                            n562 = local write "run lab01-2"(w854) -> ()
                          }
                          frame True {
                            n563 = stacked-sequence {
                              seq-local: [w867 _ _ _ _] -> [_ w891 _ _ _]
                              tunnel: w866 -> [w872 _ _ _ _]
                              tunnel: w865 -> [w869 _ _ _ _]
                              tunnel: w864 -> [w882 _ _ _ _]
                              tunnel: w863 -> [w875 _ _ _ _]
                              tunnel: w862 -> [w870 _ _ _ _]
                              tunnel: [_ w886 _ _ _] -> w861
                              tunnel: w860 -> [_ _ _ w913 _]
                              tunnel: w859 -> [_ _ _ w912 _]
                              tunnel: w858 -> [_ _ _ w911 _]
                              tunnel: w857 -> [_ _ _ _ _]
                              tunnel: w856 -> [_ _ _ _ w926]
                              frame #0 {
                                w868 = "\\"
                                n564 = local read "SET LAB01-2"() -> (w877:T5)
                                n565 = case shown="\"CYCLE TEST\"" w882 {
                                tunnel: ["L01-2-CHART TEST-" "L01-2-CYCLE TEST-" "L01-2-T-RISE TEST-"] -> w878
                                frame "CHART TEST", Default {
                                }
                                frame "CYCLE TEST" {
                                }
                                frame "T-RISE TEST" {
                                }
                                }
                                n566 = Unbundle(w877) -> ("DESCRIPTION"=w876:string)  [unwired: 4 out]
                                n567 = Concatenate Strings(w872, "\\", w870, w868, w869, w868) -> (w879:string)
                                n568 = String To Path(string=w879) -> (path=w881:path)
                                n569 = Concatenate Strings(w879, w878, w876, "-", w875, ".tdms") -> (w867:string)
                                n570 = Create Folder(path (use dialog)=w881) -> (error out=w880:errorcluster)  [unwired: 2 in, 2 out]
                                n571 = call <vilib>:"Clear Errors.vi"("error in (no error)"=w880) -> ()  [unwired: 6 in, 1 out]
                                n572 = global write "Global 1.vi" "LAB01-2 FILE"(w867) -> ()
                              }
                              frame #1 {
                                (unwired) FALSE
                                n573 = String To Path(string=w891) -> (path=w887:path)
